vi "select child.vi"(6 "wait for reply (T)":bool=TRUE, 8 "error in":errorcluster, 10 "Enum":T1=enum."PSP-603", 11 "Module ID":i32=-1) -> (0 "error out":errorcluster, 1 "timed out?":bool)   [LabVIEW 2025, in "Power Supply.lvlib"]
doc: "_____\nCreated using DQMH Framework: Event Scripter 7.1.2.1547."
uses:
  Power Supply.lvlib
  Classes/hardware-selection.ctl
  select child Argument--cluster.ctl
  select child (Reply Payload)--cluster.ctl
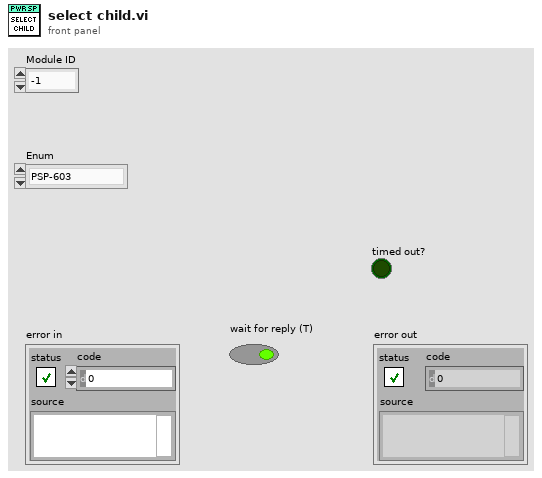
[diagram p1: front panel]
types:
  T1 = typedef "hardware-selection.ctl" = enum16{"Parent", "Simulation", "PSP-603"}
  T2 = typedef "Power Supply.lvlib/select child Argument--cluster.ctl" = cluster{"Module ID":i32, "Enum":T1, "Wait Notifier":refnum<notifier>, "wait for reply":bool}
  T3 = typedef "Power Supply.lvlib/Request Events--cluster.ctl" = cluster{"Stop Module":refnum<user-event>, "Show Panel":refnum<user-event>, "Hide Panel":refnum<user-event>, "Show Diagram":refnum<user-event>, "Get Module Execution Status":refnum<user-event>, "select child":refnum<user-event>}
  T4 = typedef "Power Supply.lvlib/select child (Reply Payload)--cluster.ctl" = cluster{"Module ID":i32, "error":errorcluster}
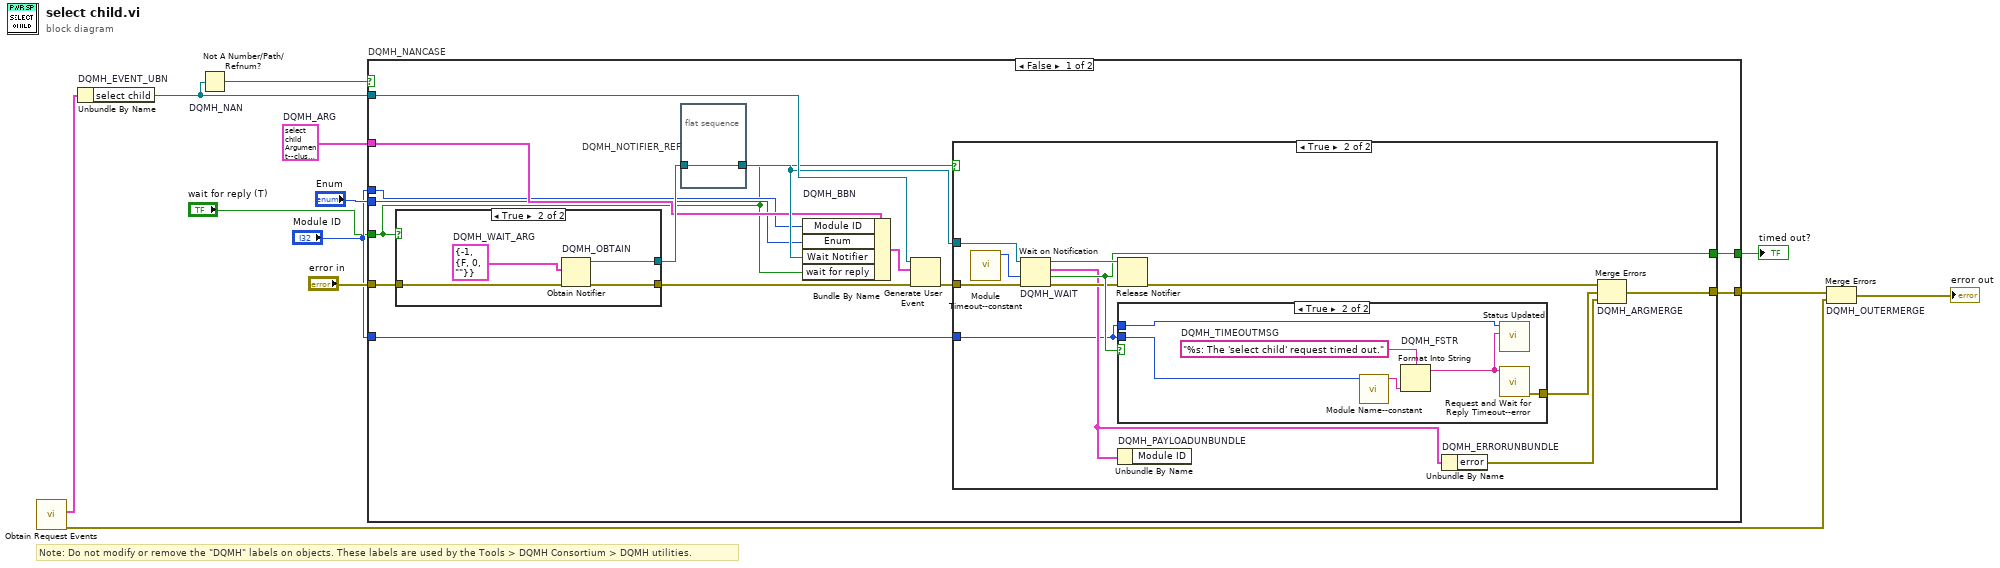
[diagram p0: block diagram]
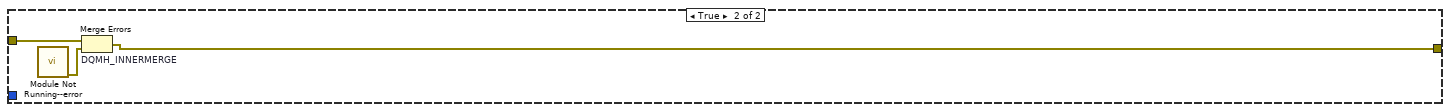
[diagram p5: hidden frame]
diagram:
  w6 = T2 {"Module ID"=-1, "Enum"=enum."PSP-603", "Wait Notifier"=refnum, "wait for reply"=FALSE}  # DQMH_ARG
  # "Note: Do not modify or remove the \"DQMH\" labels on objects. These labels are used by the Tools > DQMH Consortium > DQMH utilities."
  n1 = call "Obtain Request Events.vi"() -> ("error out"=w2:errorcluster, "Power Supply Request Events"=w1:T3)  [unwired: 10 in]
  n2 = Unbundle By Name "DQMH_EVENT_UBN"(w1) -> ("select child"=w10:refnum<user-event>)
  n3 = Not A Number/Path/Refnum? "DQMH_NAN"(number/path/refnum=w10) -> (NaN/Path/Refnum?=w9:bool)
  n4 = case "DQMH_NANCASE" shown="False" w9 {
    tunnel: "error in" -> [w26 w54]
    tunnel: w10 -> [w24 _]
    tunnel: [w21 w53] -> w7
    tunnel: [w22 _] -> w8
    tunnel: w6 -> [w17 _]
    tunnel: "Module ID" -> [w16 _]
    tunnel: "Enum" -> [w15 _]
    tunnel: "Module ID" -> [w14 _]
    tunnel: "wait for reply (T)" -> [w13 _]
    frame False {
      n5 = case shown="True" w13 {
        tunnel: w26 -> [w47 w51]
        tunnel: [w47 w50] -> w23
        tunnel: [_ w48] -> w19
        frame False {
        }
        frame True {
          w49 = T4 {"Module ID"=-1, "error"={"status"=FALSE, "code"=0, "source"=""}}  # DQMH_WAIT_ARG
          n6 = Obtain Notifier "DQMH_OBTAIN"(notification data type=w49, error in (no error)=w51) -> (notifier out=w48:refnum<notifier>, error out=w50:errorcluster)  [unwired: 2 in, 1 out]
        }
      }
      n7 = flat-sequence "DQMH_NOTIFIER_REF" {
        tunnel: w19 -> [w27]
        tunnel: [w27] -> w18
        frame #0 {
        }
      }
      n8 = Bundle By Name "DQMH_BBN"(cluster=w17, "Module ID"=w16, "Enum"=w15, "Wait Notifier"=w18, "wait for reply"=w13) -> (w20:T2)
      n9 = Generate User Event(user event=w24, event data cluster=w20, error in=w23) -> (error out=w25:errorcluster)  [unwired: 1 in, 1 out]
      n10 = case shown="True" w13 {
        tunnel: w25 -> [w28 w40]
        tunnel: w18 -> [_ w39]
        tunnel: [_ w37] -> w22
        tunnel: [w28 w36] -> w21
        tunnel: w14 -> [_ w29]
        frame False {
        }
        frame True {
          n11 = call "Module Timeout--constant.vi"() -> ("Module Timeout"=w30:i32)  [unwired: 11 in]
          n12 = Wait on Notification "DQMH_WAIT"(notifier=w39, timeout in ms (-1)=w30, error in (no error)=w40) -> (notifier out=w38:refnum<notifier>, notification=w31:T4, timed out?=w37:bool, error out=w35:errorcluster)  [unwired: 1 in]
          n13 = Release Notifier(notifier=w38, error in (no error)=w35) -> (error out=w34:errorcluster)  [unwired: 1 in, 2 out]
          n14 = case shown="True" w37 {
            tunnel: [_ w44] -> w32
            tunnel: w29 -> [_ w42]
            tunnel: w29 -> [_ w41]
            frame False {
            }
            frame True {
              w46 = "%s: The 'select child' request timed out."  # DQMH_TIMEOUTMSG
              n15 = call "Module Name--constant.vi"("Module ID"=w41) -> ("Module Name"=w43:string)  [unwired: 10 in]
              n16 = Format Into String "DQMH_FSTR"(format string=w46, w43) -> (resulting string=w45:string)  [unwired: 2 in, 1 out]
              n17 = call "Status Updated.vi"("Status"=w45, "Module ID"=w42) -> ()  [unwired: 9 in, 1 out]
              n18 = call "Request and Wait for Reply Timeout--error.vi"("Error Message"=w45) -> ("error out"=w44:errorcluster)  [unwired: 10 in]
            }
          }
          n19 = Unbundle By Name "DQMH_PAYLOADUNBUNDLE"(w31) -> ()  [unwired: 1 out]
          n20 = Unbundle By Name "DQMH_ERRORUNBUNDLE"(w31) -> ("error"=w33:errorcluster)
          n21 = Merge Errors "DQMH_ARGMERGE"(w34, w32, w33) -> (w36:errorcluster)
        }
      }
    }
    frame True {
      n22 = call "Module Not Running--error.vi"() -> ("error out"=w52:errorcluster)  [unwired: 11 in]
      n23 = Merge Errors "DQMH_INNERMERGE"(w54, w52) -> (w53:errorcluster)
    }
  }
  "timed out?" <- w8
  n24 = Merge Errors "DQMH_OUTERMERGE"(w7, w2) -> (→"error out":errorcluster)
